vi "ConsumeComma.vi"(8 "error in (no error)":errorcluster, 11 "PathTokenizer in":refnum<class "PathTokenizer.lvclass">) -> (0 "error out":errorcluster, 3 "PathTokenizer out":refnum<class "PathTokenizer.lvclass">)   [LabVIEW 2019, in "PathTokenizer.lvclass"]
uses:
  PathTokenizer.lvclass
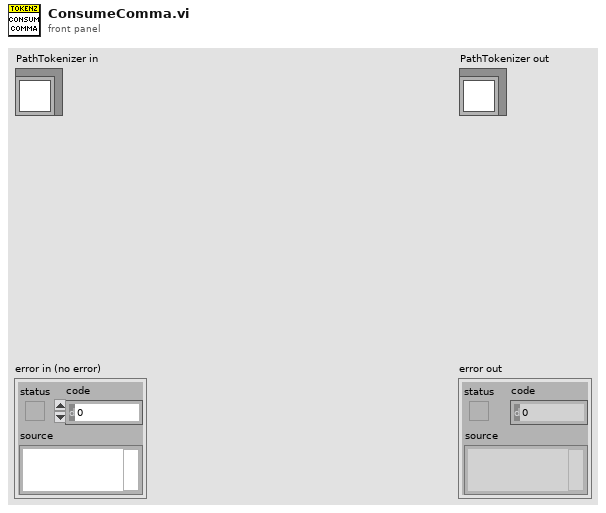
[diagram p1: front panel]
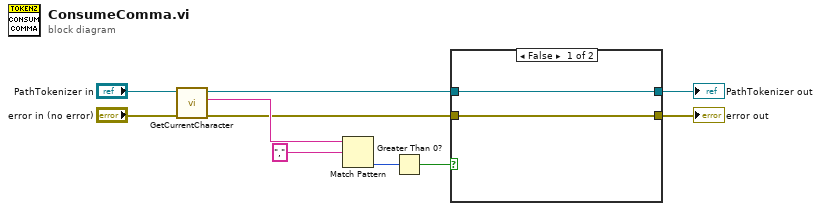
[diagram p0: block diagram]
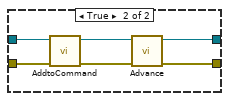
[diagram p2: hidden frame]
diagram:
  n1 = call "GetCurrentCharacter.vi"("error in (no error)"="error in (no error)", "PathTokenizer in"="PathTokenizer in") -> ("error out"=w2:errorcluster, "Current Character"=w6:string, "PathTokenizer out"=w7:refnum<class "PathTokenizer.lvclass">)  [unwired: 7 in]
  n2 = Match Pattern(string=w6, regular expression=",") -> (offset past match=w4:i32)  [unwired: 1 in, 3 out]
  n3 = Greater Than 0?(x=w4) -> (x > 0?=w1:bool)
  n4 = case shown="False" w1 {
    tunnel: w7 -> [w12 w17]
    tunnel: [w12 w16] -> w10
    tunnel: w2 -> [w11 w14]
    tunnel: [w11 w13] -> w9
    frame False {
    }
    frame True {
      n5 = call "AddtoCommand.vi"("error in (no error)"=w14, "PathTokenizer in"=w17) -> ("error out"=w15:errorcluster, "PathTokenizer out"=w18:refnum<class "PathTokenizer.lvclass">)  [unwired: 8 in]
      n6 = call "Advance.vi"("error in (no error)"=w15, "PathTokenizer in"=w18) -> ("error out"=w13:errorcluster, "PathTokenizer out"=w16:refnum<class "PathTokenizer.lvclass">)  [unwired: 8 in]
    }
  }
  "error out" <- w9
  "PathTokenizer out" <- w10
